vi "Verify Timer.vi"(8 "error in (no error)":errorcluster, 11 "State Machine in":refnum<class "State Machine.lvclass">) -> (0 "error out":errorcluster, 2 "timeout":bool, 3 "State Machine out":refnum<class "State Machine.lvclass">)   [LabVIEW 2018, in "State Machine.lvclass"]
uses:
  State Machine.lvclass
  State Machine.lvclass/State Machine.ctl
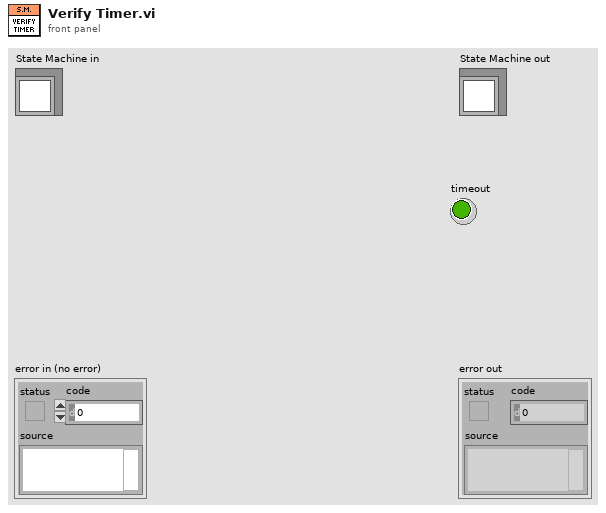
[diagram p1: front panel]
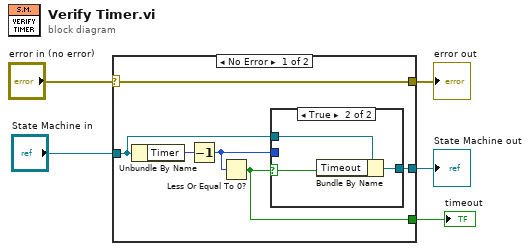
[diagram p0: block diagram]
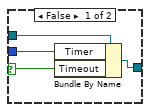
[diagram p2: hidden frame]
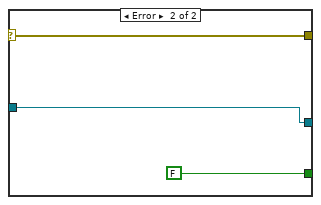
[diagram p3: hidden frame]
diagram:
  n1 = case shown="No Error" "error in (no error)" {
    selector: "error in (no error)" -> [w11 w21]
    tunnel: [w11 w21] -> w3
    tunnel: [w10 w20] -> w2
    tunnel: "State Machine in" -> [w9 w20]
    tunnel: [w6 FALSE] -> w1
    frame No Error {
      n2 = Unbundle By Name(w9) -> ("Timer"=w8:u32)
      n3 = Decrement(x=w8) -> (x-1=w7:u32)
      n4 = Less Or Equal To 0?(x=w7) -> (x <= 0?=w6:bool)
      n5 = case shown="True" w6 {
        selector: w6 -> [w12 w16]
        tunnel: [w15 w17] -> w10
        tunnel: w9 -> [w14 w18]
        tunnel: w7 -> [w13 _]
        frame False {
          n6 = Bundle By Name(cluster=w14, "Timer"=w13, "Timeout"=w12) -> (w15:refnum<class "State Machine.lvclass">)
        }
        frame True {
          n7 = Bundle By Name(cluster=w18, "Timeout"=w16) -> (w17:refnum<class "State Machine.lvclass">)
        }
      }
    }
    frame Error {
    }
  }
  "error out" <- w3
  "State Machine out" <- w2
  "timeout" <- w1
